vi "故障处理.vi"(8 "数据模式":bool, 9 "故障字典":string[][](table), 10 "原故障内容":string[](array[string]), 11 "故障信息":string[](array[string])) -> (3 "故障内容":string[](array[string]))   [LabVIEW 2021]
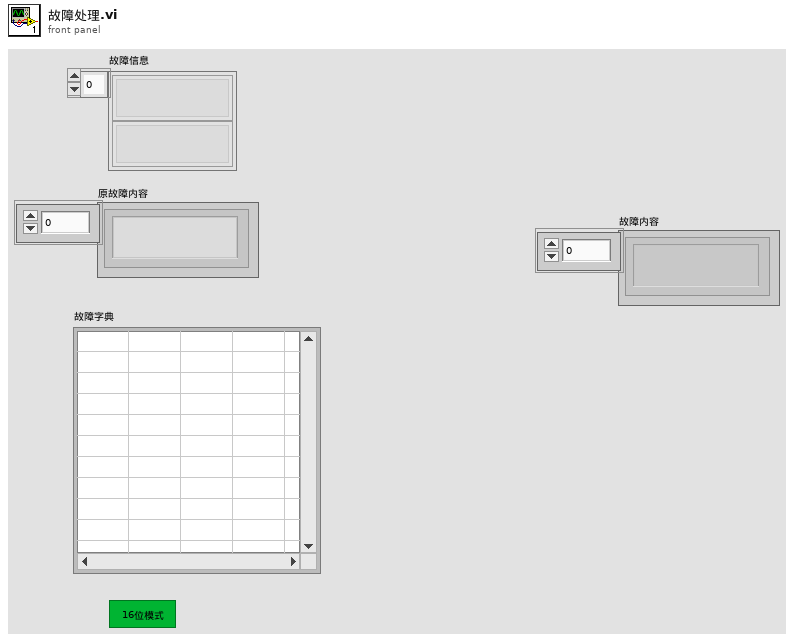
[diagram p1: front panel]
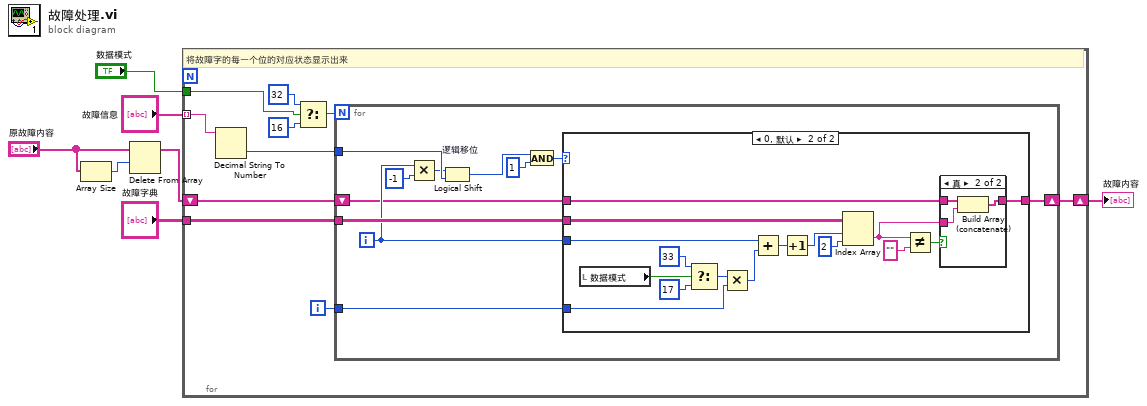
[diagram p0: block diagram]
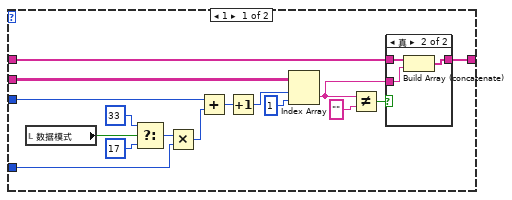
[diagram p2: hidden frame]
diagram:
  n1 = Array Size(array="原故障内容") -> (size(s)=w7:i32)
  n2 = Delete From Array(array="原故障内容", length=w7) -> (array with subset deleted=w6:string[])  [unwired: 1 in, 1 out]
  n3 = for "For循环" {
    tunnel: "故障信息" -> [w17] mode=indexing
    tunnel: "故障字典" -> [w16]
    shift-right: [w13] -> w5
    shift-left: w6 -> [w14]
    tunnel: "数据模式" -> [w8]
    i -> [w15]
    # "将故障字的每一个位的对应状态显示出来"
    n4 = Decimal String To Number(string=w17) -> (number=w12:i32)  [unwired: 2 in, 1 out]
    n5 = Select(t=32, s=w8, f=16) -> (s? t:f=w9:i32)
    n6 = for "For循环" {
      N: w9 -> [_]
      tunnel: w12 -> [w28]
      tunnel: w16 -> [w24]
      tunnel: w15 -> [w23]
      shift-right: [w18] -> w13
      shift-left: w14 -> [w19]
      i -> [w22]
      n7 = Multiply(x=w22, y=-1) -> (x*y=w26:i32)
      n8 = Logical Shift "逻辑移位"(y=w26, x=w28) -> (x << y=w20:i32)
      n9 = And(x=w20, y=1) -> (x .and. y?=w25:i32)
      n10 = case shown="0, 默认" w25 {
        tunnel: w24 -> [w44 w64]
        tunnel: w23 -> [w42 w62]
        tunnel: w22 -> [w40 w60]
        tunnel: w19 -> [w37 w57]
        tunnel: [w36 w56] -> w18
        frame 1 {
          n11 = local read "数据模式"() -> (w31:bool)
          n12 = Select(t=33, s=w31, f=17) -> (s? t:f=w29:i32)
          n13 = Multiply(x=w29, y=w42) -> (x*y=w41:i32)
          n14 = Add(x=w40, y=w41) -> (x+y=w39:i32)
          n15 = Increment(x=w39) -> (x+1=w38:i32)
          n16 = Index Array(array=w44, index (row)=w38, index (col)=1 ("禁用的索引 (列)")) -> (element=w34:string)
          n17 = Not Equal?(x=w34, y="") -> (x != y?=w33:bool)
          n18 = case shown="真" w33 {
            tunnel: w37 -> [w45 w48]
            tunnel: [w45 w47] -> w36
            tunnel: w34 -> [_ w46]
            frame False {
            }
            frame True {
              n19 = Build Array (concatenate)(w48, w46) -> (w47:string[])
            }
          }
        }
        frame 0, Default {
          n20 = local read "数据模式"() -> (w51:bool)
          n21 = Select(t=33, s=w51, f=17) -> (s? t:f=w49:i32)
          n22 = Multiply(x=w49, y=w62) -> (x*y=w61:i32)
          n23 = Add(x=w60, y=w61) -> (x+y=w59:i32)
          n24 = Increment(x=w59) -> (x+1=w58:i32)
          n25 = Index Array(array=w64, index (row)=w58, index (col)=2 ("禁用的索引 (列)")) -> (element=w54:string)
          n26 = Not Equal?(x=w54, y="") -> (x != y?=w53:bool)
          n27 = case shown="真" w53 {
            tunnel: w57 -> [w65 w68]
            tunnel: [w65 w67] -> w56
            tunnel: w54 -> [_ w66]
            frame False {
            }
            frame True {
              n28 = Build Array (concatenate)(w68, w66) -> (w67:string[])
            }
          }
        }
      }
    }
  }
  "故障内容" <- w5
